vi "Read Config (with defaults).vi"(8 "error in (no error)":errorcluster) -> (0 "error out":errorcluster, 3 "Settings out":T1 {"Resistance Parameters"."Stop Bits (10: 1 bit)" items=["1.0"=10, "1.5"=15, "2.0"=20]; "Resistance Parameters"."Data Bits (8)" min=5 max=8 step=1; "Resistance Parameters"."Flow Control (none)" items=["None", "XON/XOFF", "RTS/CTS", "XON/XOFF & RTS/CTS", "DTR/DSR", "XON/XOFF & DTR/DSR"]; "Crank Motor Parameters"."flow control (none)" items=["None", "XON/XOFF", "RTS/CTS", "XON/XOFF & RTS/CTS", "DTR/DSR", "XON/XOFF & DTR/DSR"]; "Crank Motor Parameters"."parity (even)" items=["None", "Odd", "Even", "Mark", "Space"]; "Sequence"."Steady State Max Wait (s)" format="%.2g"; "Sequence"."Steady State Window (s)" format="%.2g"; "Sequence"."Steady State +/-RPM" format="%.2g"})   [LabVIEW 2021, in "Config Module.lvlib"]
uses:
  Config Module.lvlib
  Controls/Config File Operation Enum.ctl
  Logging/Logging Configuration.ctl
  Logging/Logging.lvlib
  Settings/Sequence Cluster.ctl
  controls/CSV Log Cluster.ctl
  Peloton Bike/Signal Type.ctl
  Peloton Bike/Bike Parameters.ctl
  Crank Motor/Signal Type.ctl
  Crank Motor/Crank Motor Parameters.ctl
  Resistance Motor/Signal Type.ctl
  Resistance Motor/Resistance Motor Default Params.ctl
  Resistance Motor/Resistance Parameters.ctl
  Acquisition/Signal Type.ctl
  Acquisition/Acquisition Parameters.ctl
  Settings/Settings.ctl
  Settings/Settings.lvlib
panel:
  # "Steady State when"
  # "RPM is within"
  # "RPM of set RPM for last"
  # "seconds"
  # "OR"
  # "seconds since last step change"
  # "More than"
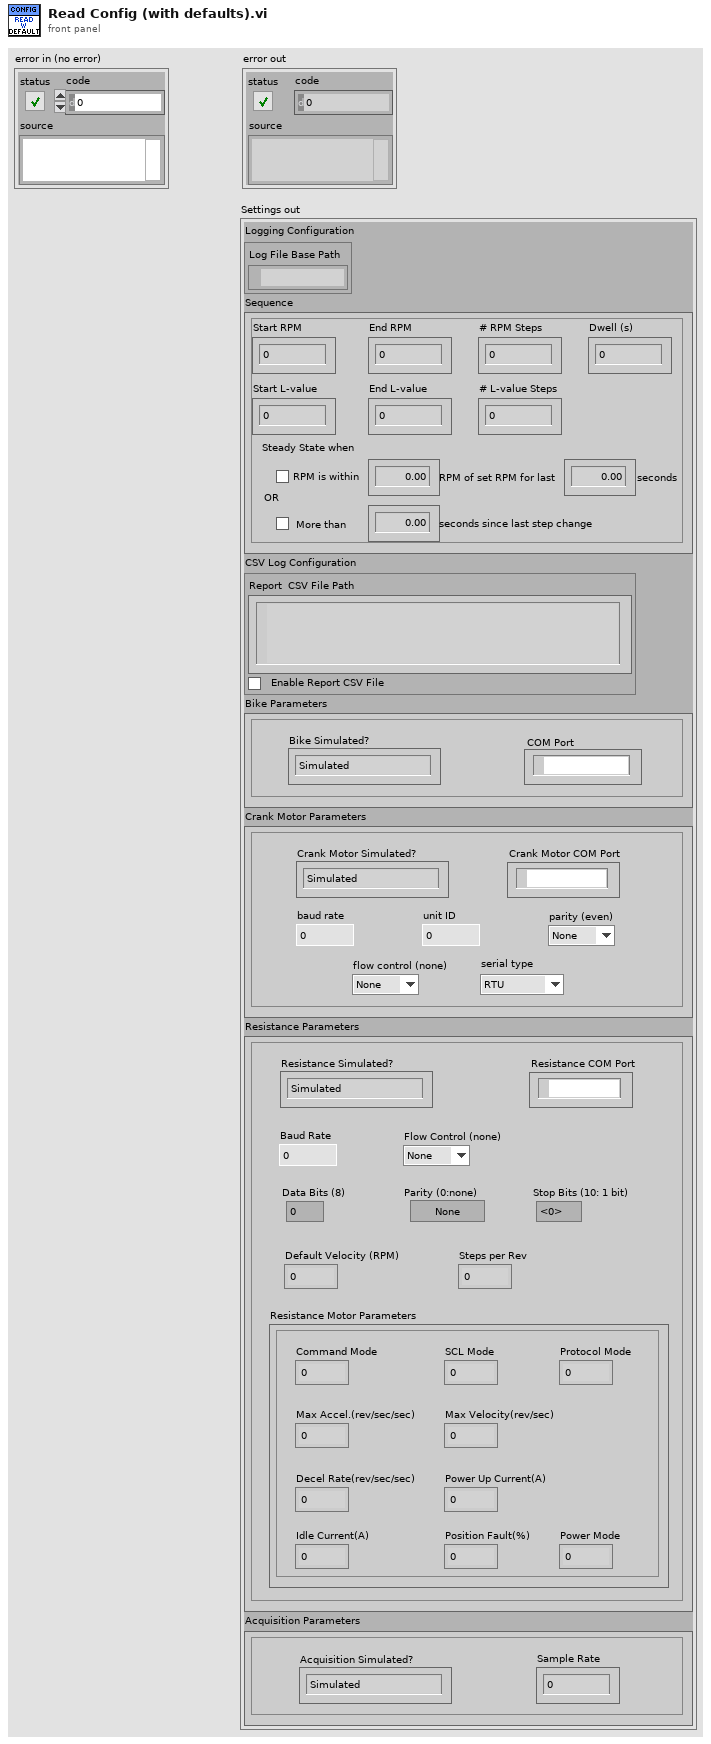
[diagram p1: front panel]
types:
  T1 = typedef "Settings.lvlib/Settings.ctl" = cluster{"Logging Configuration":T2, "Sequence":T3, "CSV Log Configuration":T4, "Bike Parameters":T5, "Crank Motor Parameters":T7, "Resistance Parameters":T9, "Acquisition Parameters":T12}
  T2 = typedef "Logging.lvlib/Logging Configuration.ctl" = cluster{"Log File Base Path":path}
  T3 = typedef "Sequence Cluster.ctl" = cluster{"Start RPM":dbl, "End RPM":dbl, "# RPM Steps":i32, "Dwell (s)":dbl, "Start L-value":i32, "End L-value":i32, "# L-value Steps":i32, "Steady State +/-RPM":dbl, "Enable Steady State +/- RPM":bool, "Steady State Window (s)":dbl, "Enable Steady State Max Wait":bool, "Steady State Max Wait (s)":dbl}
  T4 = typedef "CSV Log Cluster.ctl" = cluster{"Report  CSV File Path":path, "Enable Report CSV File":bool}
  T5 = typedef "Bike Parameters.ctl" = cluster{"Bike Simulated?":T6, "COM Port":refnum<visa-resource-name>}
  T6 = typedef "Peloton Bike.lvlib/Signal Type.ctl" = enum16{"Simulated", "Real"}
  T7 = typedef "Crank Motor Parameters.ctl" = cluster{"Crank Motor COM Port":refnum<visa-resource-name>, "baud rate":u32, "unit ID":u8, "parity (even)":u16, "flow control (none)":u16, "serial type":enum16{"RTU", "ASCII"}, "Crank Motor Simulated?":T8}
  T8 = typedef "Crank Motor.lvlib/Signal Type.ctl" = enum16{"Simulated", "Real"}
  T9 = typedef "Resistance Parameters.ctl" = cluster{"Resistance Simulated?":T10, "Resistance COM Port":refnum<visa-resource-name>, "Baud Rate":u32, "Flow Control (none)":u16, "Default Velocity (RPM)":dbl, "Steps per Rev":i32, "Data Bits (8)":u16, "Parity (0:none)":enum16{"None", "Odd", "Even", "Mark", "Space"}, "Stop Bits (10: 1 bit)":u16, "Resistance Motor Parameters":T11}
  T10 = typedef "Resistance Motor.lvlib/Signal Type.ctl" = enum16{"Simulated", "Real"}
  T11 = typedef "Resistance Motor Default Params.ctl" = cluster{"Command Mode":u16, "SCL Mode":u16, "Protocol Mode":u16, "Max Accel.(rev/sec/sec)":u16, "Max Velocity(rev/sec)":u16, "Decel Rate(rev/sec/sec)":u16, "Power Up Current(A)":u16, "Idle Current(A)":u16, "Position Fault(%)":u16, "Power Mode":u16}
  T12 = typedef "Acquisition.lvlib/Acquisition Parameters.ctl" = cluster{"Acquisition Simulated?":T13, "Sample Rate":dbl}
  T13 = typedef "Acquisition.lvlib/Signal Type.ctl" = enum16{"Simulated", "Real"}
  T14 = typedef "Config Module.lvlib/Config File Operation Enum.ctl" = enum16{"Read", "Write"}
  T15 = typedef "Config Module.lvlib/Main Config Cluster.ctl" = cluster{"Notebook":string, "OPC Module Configs":T16[], "Feed Module Configs":T26[], "Log File Path":path, "TT Module Configs":T46[], "DAQ Config":T47, "PT Module Configs":T49[], "Scale Module Configs":T50[], "Pump Module Configs":T52[], "U3 Module Configs":T54[], "Decoration Module Configs":T55[], "Flow Module Configs":T56[], "TCU Module Configs":T58[], "Steps":T66, "Abort":bool, "DO Module Configs":T68[], "PR Module Configs":T73[], "SC Module Configs":T77[], "AM Module Configs":T80[], "CM Module Configs":T83[], "Cycle Period":dbl}
  T16 = typedef "OPC UA.lvlib/OPC Module Config.ctl" = cluster{"State":T17, "GUID":string, "Process Name":string, "User name":string, "Drop Coords":T18, "Configuration":T19, "First Iteration":bool, "Data":cluster{"Object Name":string, "Variable Array":T20[]}[], "Load Count":i32, "Log Started":bool, "subscription ID out":T23, "OPC UA client refnum out":T24, "Event Registration Refnum":refnum<event-registration>, "Start Time":timestamp, "Current Time":timestamp, "Tag Data":T25[]}
  T17 = typedef "Scale Module.lvlib/Scale Module Engine.lvlib/State Enum.ctl" = enum16{"Measuring", "Idle"}
  T18 = typedef "LVPoint32TypeDef.ctl" = cluster{"Horizontal":i32, "Vertical":i32}
  T19 = typedef "OPC UA.lvlib/OPC Settings.ctl" = cluster{"Cycle Period":dbl, "server endpoint URL":string, "security policy":cluster{"message mode":enum16{"None", "Sign", "Sign and Encrypt"}, "security":enum16{"Basic256", "Basic128Rsa15"}}, "Trust Any Server":bool}
  T20 = typedef "OPC UA.lvlib/Variable Data Cluster.ctl" = cluster{"node ID":T21, "browse name":string, "status":T22, "timestamp":timestamp, "value ":variant}
  T21 = typedef "NodeId.ctl" = string
  T22 = typedef "OPC UA StatusCode.ctl" = u32
  T23 = typedef "Subscription ID.ctl" = u32
  T24 = typedef "OPC UA Client Refnum.ctl" = refnum<k21>
  T25 = typedef "OPC UA.lvlib/OPC Tag Data.ctl" = cluster{"Include this Device":bool, "Device Name":string, "OPC Tag Data":cluster{"Tag":string, "Value":variant, "Time Stamp":timestamp}[]}
  T26 = typedef "Feed Module.lvlib/Feed Module Config Cluster.ctl" = cluster{"GUID":string, "Drop Coords":T18, "Process Name":string, "User name":string, "Queue Name":string, "Settings":T27, "Settings Load Count":i32, "OP Load Count":i32}
  T27 = typedef "Feed Module.lvlib/Feed Module Settings Cluster.ctl" = cluster{"Cycle Period":dbl, "Ismatech":T28, "Masterflex":T29, "Mettler":T30, "Bronkhorst M13 Flow Meter":T31, "PID 2 Parameters":T32, "Manual Entry":dbl, "Auto?":bool, "PID range":cluster{"PID High":dbl, "PID Low":dbl, "High Warning":dbl}, "Tacmina Settings":T35, "KNF SIMDOS Settings":T36, "ASIA Pump C":T37, "VICI Settings":T38, "FLOM Settings":T39, "SSI PR/LD Settings":T40, "Masterflex 75211 Settings":T41, "SSI P40 Settings":T42, "Ismatech 3 Channel Settings":T43, "Bronkhorst M14 Settings":T44, "Reset Totalizer":bool, "Input Num Alarm Settings":T45[], "Control Type":enum32{"g/min", "ml/min"}, "Front End Display Options":cluster{"Temperature":bool, "Scale Grams":bool, "Density":bool, "Flow (g/min)":bool, "Flow (ml/min)":bool, "PSIG":bool, "Total Grams":bool, "Updated":bool}}
  T28 = typedef "Ismatec ISM 831C.lvlib/Ismatech ISM831C Settings Cluster.ctl" = cluster{"VISA resource name":refnum<visa-resource-name>, "Simulated?":bool, "Pump Number":dbl, "Reverse?":bool}
  T29 = typedef "Masterflex 7550-30.lvlib/Settings Cluster.ctl" = cluster{"VISA resource name":refnum<visa-resource-name>, "Simulated?":bool, "Pump Number":dbl, "Reverse?":bool}
  T30 = typedef "Mettler Toledo.lvlib/Settings Cluster.ctl" = cluster{"VISA resource name":refnum<visa-resource-name>, "Simulated?":bool}
  T31 = typedef "Bronkhorst M13 Flow Meter.lvlib/Settings Cluster.ctl" = cluster{"VISA resource name":refnum<visa-resource-name>, "Simulated?":bool, "Smoothing Steps":i32}
  T32 = typedef "PID 2 Parameters Cluster.ctl" = cluster{"Input Device":T33, "Output Device":T34, "Setpoint":dbl, "PID gains":cluster{"proportional gain (Kc)":dbl, "integral time (Ti, min)":dbl, "derivative time (Td, min)":dbl}}
  T33 = typedef "PID Input Enum.ctl" = enum16{"Default", "Bronkhorst M13", "Bronkhorst M14", "Scale Rate of Change"}
  T34 = typedef "PID 2 Output Enum.ctl" = enum16{"Default", "Ismatec ISM 4308", "Ismatec ISM 831C", "Masterflex 7550-30", "VICI M6", "VICI M50", "Tacmina QI", "KNF SIMDOS", "ASIA Type C", "FLOM UI-22-11", "SSI PR/LD", "SSI P40", "Masterflex 75211-70"}
  T35 = typedef "Tacmina QI.lvlib/Tacmina QI DAQ Setting.ctl" = cluster{"Analog DAQ Task":refnum<k21>, "Digital DAQ Task":refnum<k21>}
  T36 = typedef "KNF SIMDOS.lvlib/Settings Cluster plus SIMDOS.ctl" = cluster{"VISA resource name":refnum<visa-resource-name>, "Simulated?":bool}
  T37 = typedef "ASIA Pump.lvlib/Pump Settings.ctl" = cluster{"ASIA Pump #":i32, "channel":i32, "Simulated":bool}
  T38 = typedef "VICI M6 M50 Party Mode.lvlib/Settings Cluster.ctl" = cluster{"VISA resource name":refnum<visa-resource-name>, "Pump ID":string, "Pump Head Vol":dbl, "Reverse?":bool, "Simulated?":bool}
  T39 = typedef "FLOM Pump.lvlib/Settings Cluster.ctl" = cluster{"VISA resource name":refnum<visa-resource-name>, "Simulated?":bool, "Pump Number":dbl}
  T40 = typedef "SSI PR or LD Pump.lvlib/SSI PR or LD Settings Cluster.ctl" = cluster{"VISA resource name":refnum<visa-resource-name>, "Simulated?":bool}
  T41 = typedef "Masterflex 75211.lvlib/Masterflex 75211 DAQ Setting.ctl" = cluster{"Analog DAQ Task":refnum<k21>, "Digital DAQ Task":refnum<k21>}
  T42 = typedef "SSI P40 Pump.lvlib/SSI P40 Settings Cluster.ctl" = cluster{"VISA resource name":refnum<visa-resource-name>, "Simulated?":bool}
  T43 = typedef "Ismatec 4308.lvlib/Ismatec 4083.ctl" = cluster{"VISA resource name":refnum<visa-resource-name>, "Pump Number":i16, "Channel Number":i16, "Simulated?":bool, "Reverse?":bool}
  T44 = typedef "Bronkhorst M14 Flow Meter.lvlib/Settings Cluster.ctl" = cluster{"VISA resource name":refnum<visa-resource-name>, "Simulated?":bool, "Smoothing Steps":i32}
  T45 = typedef "Numeric Alarm Settings Cluster.ctl" = cluster{"enable? (F)":bool, "name":string, "alarm type":enum16{"HI_HI", "HI", "LO", "LO_LO"}, "level/change":dbl, "deadband/time":dbl, "alarm delay":dbl, "priority":u32, "ack type":enum16{"Auto", "User", "None", "Each Occurrence"}, "area":string, "description":string, "log? (T)":bool}
  T46 = typedef "TT Module.lvlib/TT Module Config Cluster.ctl" = cluster{"GUID":string, "Drop Coords":T18, "Input Channel Tag Name ":string, "Process Name":string, "User name":string, "Queue Name":string, "Input Channel Numeric Alarm Settings":T45[]}
  T47 = typedef "DAQ.lvlib/Hardware Configuration.ctl" = cluster{"Tasks Array":T48[]}
  T48 = typedef "Task Cluster.ctl" = cluster{"DAQmx Task":refnum<k21>, "Read-Write Radio":enum32{"Read", "Write"}}
  T49 = typedef "PT Module.lvlib/PT Module Config Cluster.ctl" = cluster{"GUID":string, "Drop Coords":T18, "Input Channel Tag Name ":string, "Process Name":string, "User name":string, "Queue Name":string, "Input Channel Numeric Alarm Settings":T45[]}
  T50 = typedef "Scale Module.lvlib/Scale Module Config Cluster.ctl" = cluster{"GUID":string, "Drop Coords":T18, "Process Name":string, "User name":string, "Queue Name":string, "Settings":T51, "Load Count":i32}
  T51 = typedef "Scale Module.lvlib/Scale Module Settings Cluster.ctl" = cluster{"Cycle Period":dbl, "Mettler":T30, "Scale Type":string}
  T52 = typedef "Pump Module.lvlib/Pump Module Config Cluster.ctl" = cluster{"GUID":string, "Drop Coords":T18, "Process Name":string, "User name":string, "Queue Name":string, "Settings":T53, "Load Count":i32}
  T53 = typedef "Pump Module.lvlib/Pump Module Settings Cluster.ctl" = cluster{"Cycle Period":dbl, "Manual Entry":dbl, "Output Device":T34, "Ismatech":T28, "Ismatech 3 Channel Settings":T43, "Masterflex":T29, "VICI Settings":T38, "Tacmina Settings":T35, "KNF SIMDOS Settings":T36, "ASIA Pump C":T37, "FLOM Settings":T39, "SSI PR/LD Settings":T40, "SSI P40 Settings":T40, "Masterflex 75211 Settings":T41, "Pump Calibration File":path, "Calibration Slope":dbl, "Calibration Y Intercept":dbl, "Pump Cal Enum":u16, "Reset Totalizer":bool}
  T54 = typedef "U3 Module.lvlib/U3 Module Config Cluster.ctl" = cluster{"GUID":string, "Drop Coords":T18, "AI Channel Number":enum16{"Default", "AI0", "AI1", "AI2", "AI3", "AI4", "AI5", "AI6", "AI7"}, "Process Name":string, "User name":string, "Queue Name":string, "Input Channel Numeric Alarm Settings":T45[]}
  T55 = typedef "Decoration Module Config Cluster.ctl" = cluster{"GUID":string, "Drop Coords":T18, "Decoration Filepath":path}
  T56 = typedef "Flow Module.lvlib/Flow Module Config Cluster.ctl" = cluster{"GUID":string, "Drop Coords":T18, "Process Name":string, "User name":string, "Queue Name":string, "Settings":T57, "Load Count":i32}
  T57 = typedef "Flow Module.lvlib/Flow Module Settings Cluster.ctl" = cluster{"Cycle Period":dbl, "Flow Meter Type":string, "Bronkhorst M13 Settings":T31, "Bronkhorst M14 Settings":T44, "Reset Totalizer":bool}
  T58 = typedef "TCU Module.lvlib/TCU Module Config Cluster.ctl" = cluster{"GUID":string, "Drop Coords":T18, "Process Name":string, "User name":string, "Queue Name":string, "Settings":T59, "Load Count":i32, "Power Level Changed":bool}
  T59 = typedef "TCU Module.lvlib/TCU Module Settings Cluster.ctl" = cluster{"Cycle Period":dbl, "Setpoint Entry":dbl, "Output Device":T60, "Huber Ministat 230 Settings":T61, "Lauda Settings":T62, "Julabo FP-50 Settings":T63, "Internal Control?":bool, "Huber Unistat 410 Settings":T64, "HOTCOIL Settings":T65}
  T60 = typedef "Output Devices.ctl" = enum16{"Default", "Huber Ministat 230", "Huber Unistat 410", "Lauda XT-150", "Julabo FP-50", "HotCoil"}
  T61 = typedef "Huber Ministat 230 TCU.lvlib/Huber Settings.ctl" = cluster{"VISA resource name":refnum<visa-resource-name>, "Simulated?":bool}
  T62 = typedef "Lauda TCU.lvlib/Lauda Settings.ctl" = cluster{"VISA resource name":refnum<visa-resource-name>, "Simulated?":bool, "Pump Power":i32}
  T63 = typedef "Julabo Type FP-50 TCU.lvlib/Julabo FP-50 Settings.ctl" = cluster{"VISA resource name":refnum<visa-resource-name>, "Simulated?":bool, "Pump Power":i32}
  T64 = typedef "Huber Unistat 410 TCU.lvlib/Huber Unistat 410 RS485 Settings.ctl" = cluster{"VISA resource name":refnum<visa-resource-name>, "Address":i8, "Simulated?":bool}
  T65 = typedef "HotCoil.lvlib/HotCoil Settings.ctl" = cluster{"VISA resource name":refnum<visa-resource-name>, "Simulated?":bool}
  T66 = typedef "Not Sure Where this is Used.ctl" = T67[]
  T67 = typedef "Sequencing Library.lvlib/Squence Control.ctl" = cluster{"Module":string, "Control":u16, "Value":dbl, "Wait (sec)":dbl}
  T68 = typedef "D-O Module.lvlib/D-O Module Config Cluster.ctl" = cluster{"GUID":string, "Drop Coords":T18, "Process Name":string, "User name":string, "Queue Name":string, "Settings":T69, "Load Count":i32}
  T69 = typedef "D-O Module.lvlib/Valve Clusters.ctl" = cluster{"Valve Settings":T70, "Valve Type":enum16{"Default", "Digital Output Valve", "VICI Electronic Actuator"}, "Time On (Sec)":dbl, "Time Off (Sec)":dbl, "Run?":bool}
  T70 = typedef "D-O Module.lvlib/D-O Module Settings Cluster.ctl" = cluster{"D-O Settings":T71, "VICI Electronic Actuator":T72}
  T71 = typedef "D-O Module.lvlib/D-O Device Settings Cluster.ctl" = cluster{"DAQmx Task Name":refnum<k21>, "Output Channel":u16, "Output Channel Names":string[]}
  T72 = typedef "VICI Electronic Actuator.lvlib/VICI Electronic Actuator Settings.ctl" = cluster{"VISA resource name":refnum<visa-resource-name>, "Mode":enum16{"Two Positions With Stops", "Two Positions Without Stops", "Mutiposition"}, "Simulated":bool}
  T73 = typedef "4-20mA Module.lvlib/4-20mA Module Config Cluster.ctl" = cluster{"GUID":string, "Drop Coords":T18, "Process Name":string, "User name":string, "Queue Name":string, "Settings":T74, "Settings Load Count":i32}
  T74 = typedef "4-20mA Module.lvlib/4-20mA Module Settings Cluster.ctl" = cluster{"Cycle Period":dbl, "PID 2 Parameters":cluster{"Input Device":enum16{"Default", "4-20mA"}, "Output Device":enum16{"Default", "Equilibar Pressure Reg", "Flow Regulator"}, "Setpoint":dbl, "PID gains":cluster{"proportional gain (Kc)":dbl, "integral time (Ti, min)":dbl, "derivative time (Td, min)":dbl}, "output range":cluster{"output low":dbl, "output high":dbl}}, "Manual Entry":dbl, "Auto?":bool, "4-20mA Input Settings":T75, "4-20mA Out Settings":T76, "Input Channel Tag Name ":string}
  T75 = typedef "Pressure Transmitter Library.lvlib/Pressure Transmitter Device Settings.ctl" = cluster{"Input Channel ":u16}
  T76 = typedef "Pressure Regulator Library.lvlib/Pressure Regulator Device Settings.ctl" = cluster{"Output DAQ Task":refnum<k21>}
  T77 = typedef "Sonicator Module.lvlib/Sonicator Module Config Cluster.ctl" = cluster{"GUID":string, "Drop Coords":T18, "Process Name":string, "User name":string, "Queue Name":string, "Settings":T78, "Load Count":i32}
  T78 = typedef "Sonicator Module.lvlib/Sonicator Module Settings Cluster.ctl" = cluster{"Cycle Period":dbl, "Sonicator Type":string, "SS P100 Settings":T79, "Setpoint (µm)":dbl, "Cutoff (W)":dbl}
  T79 = typedef "Sonic Systems P100.lvlib/Sonic Systems P100 Settings.ctl" = cluster{"VISA resource name":refnum<visa-resource-name>, "Simulated?":bool}
  T80 = typedef "Agitator Module.lvlib/Agitator Module Config Cluster.ctl" = cluster{"GUID":string, "Drop Coords":T18, "Process Name":string, "User name":string, "Queue Name":string, "Settings":T81, "Load Count":i32}
  T81 = typedef "Agitator Module.lvlib/Agitator Module Settings Cluster.ctl" = cluster{"Cycle Period":dbl, "Agitator Type":string, "Setpoint (µm)":dbl, "IKA EUROSTAR Settings":T82}
  T82 = typedef "IKA EUROSTAR.lvlib/IKA EUROSTAR Settings.ctl" = cluster{"VISA resource name":refnum<visa-resource-name>, "Simulated?":bool}
  T83 = typedef "Centrifuge Module.lvlib/Centrifuge Module Config Cluster.ctl" = cluster{"GUID":string, "Drop Coords":T18, "Process Name":string, "User name":string, "Queue Name":string, "Settings":T84, "Load Count":i32}
  T84 = typedef "Centrifuge Module.lvlib/Centrifuge Module Settings Cluster.ctl" = cluster{"Cycle Period":dbl, "Manual Entry":dbl, "Output Device":T85, "EPOS4 Settings":T86}
  T85 = typedef "Device Selection.ctl" = enum16{"Default", "EPOS4"}
  T86 = typedef "EPOS4.lvlib/EPOS Communication Settings.ctl" = cluster{"VISA resource name":refnum<visa-resource-name>, "axis":cluster{"keyHandle":u32, "nodeId":u16}, "Simulated?":bool}
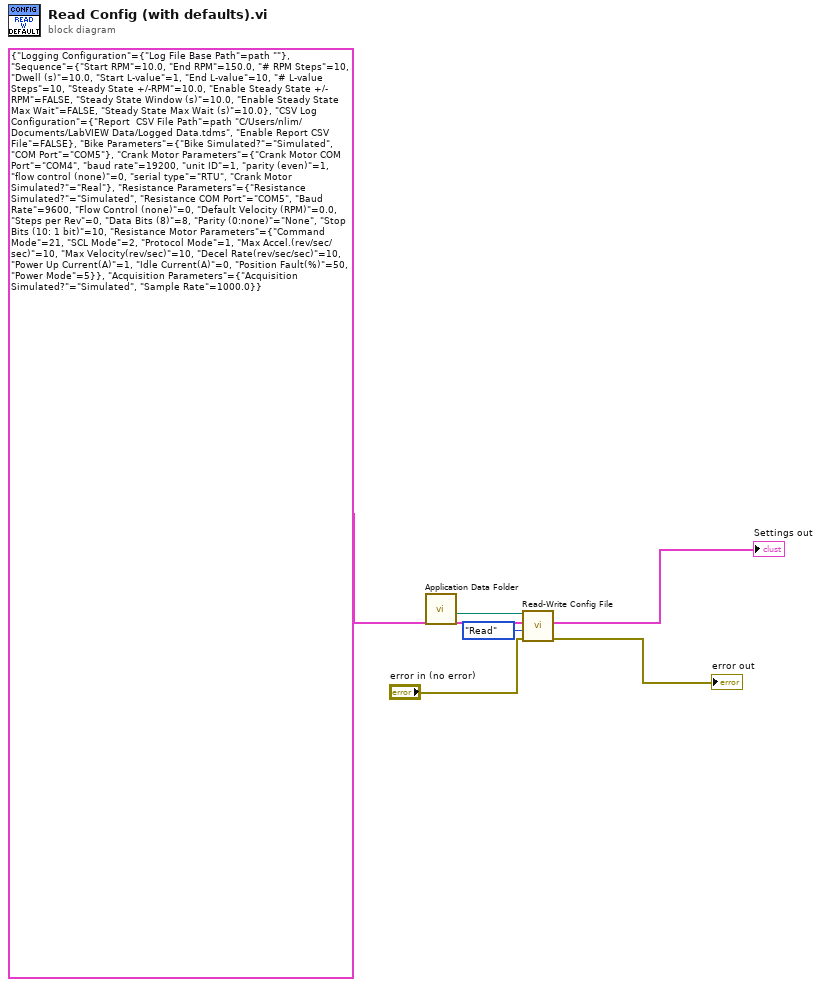
[diagram p0: block diagram]
diagram:
  n1 = call "Application Data Folder.vi"() -> ("Config Filepath"=w6:path)  [unwired: 7 in, 4 out]
  n2 = call "Read-Write Config File.vi"("configuration file path"=w6, "Main Config in"=T1 {"Logging Configuration"={"Log File Base Path"=path ""}, "Sequence"={"Start RPM"=10.0, "End RPM"=150.0, "# RPM Steps"=10, "Dwell (s)"=10.0, "Start L-value"=1, "End L-value"=10, "# L-value Steps"=10, "Steady State +/-RPM"=10.0, "Enable Steady State +/- RPM"=FALSE, "Steady State Window (s)"=10.0, "Enable Steady State Max Wait"=FALSE, "Steady State Max Wait (s)"=10.0}, "CSV Log Configuration"={"Report  CSV File Path"=path "C:/Users/nlim/Documents/LabVIEW Data/Logged Data.tdms", "Enable Report CSV File"=FALSE}, "Bike Parameters"={"Bike Simulated?"=enum."Simulated", "COM Port"="COM5"}, "Crank Motor Parameters"={"Crank Motor COM Port"="COM4", "baud rate"=19200, "unit ID"=1, "parity (even)"=1, "flow control (none)"=0, "serial type"=enum."RTU", "Crank Motor Simulated?"=enum."Real"}, "Resistance Parameters"={"Resistance Simulated?"=enum."Simulated", "Resistance COM Port"="COM5", "Baud Rate"=9600, "Flow Control (none)"=0, "Default Velocity (RPM)"=0.0, "Steps per Rev"=0, "Data Bits (8)"=8, "Parity (0:none)"=enum."None", "Stop Bits (10: 1 bit)"=10, "Resistance Motor Parameters"={"Command Mode"=21, "SCL Mode"=2, "Protocol Mode"=1, "Max Accel.(rev/sec/sec)"=10, "Max Velocity(rev/sec)"=10, "Decel Rate(rev/sec/sec)"=10, "Power Up Current(A)"=1, "Idle Current(A)"=0, "Position Fault(%)"=50, "Power Mode"=5}}, "Acquisition Parameters"={"Acquisition Simulated?"=enum."Simulated", "Sample Rate"=1000.0}} ("Settings in"), "Mode"=Config_File_Operation_Enum."Read", "error in"="error in (no error)") -> ("Main Config out"=→"Settings out":T15, "error out"=→"error out":errorcluster)  [unwired: 4 in, 1 out]
